vi "cam_polar.vi"(0 "camera values":T1, 2 "points":cluster{"x-point":dbl, "y-point":dbl}[](array[cluster]), 3 "camera height":sgl, 4 "Color Code":dbl) -> (6 "points polar":cluster{"degrees right":dbl, "distance":dbl}[](array[cluster]) {"degrees right" format="%#_6f"}, 7 "Angle and color of Buoys":dbl[][](array[numeric]))   [LabVIEW 2018]
panel:
  out "Array":dbl[](array[numeric])
  in  "camera angle":dbl
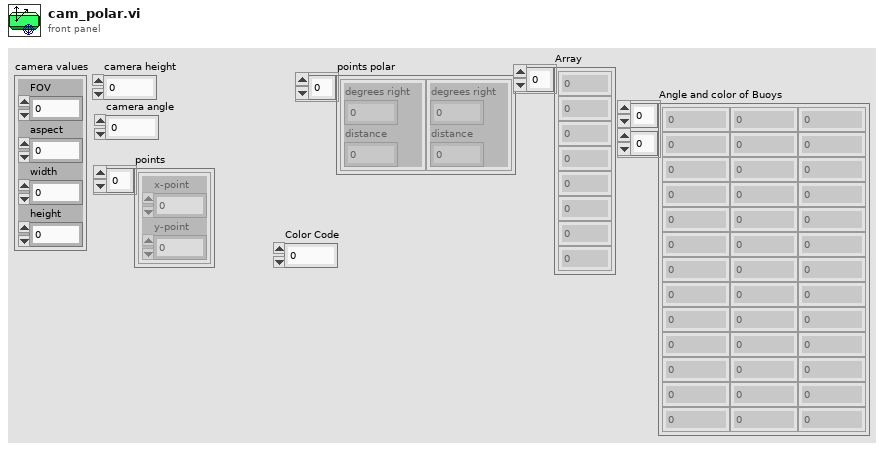
[diagram p1: front panel]
types:
  T1 = cluster{"FOV":dbl, "aspect":dbl, "width":dbl, "height":dbl}
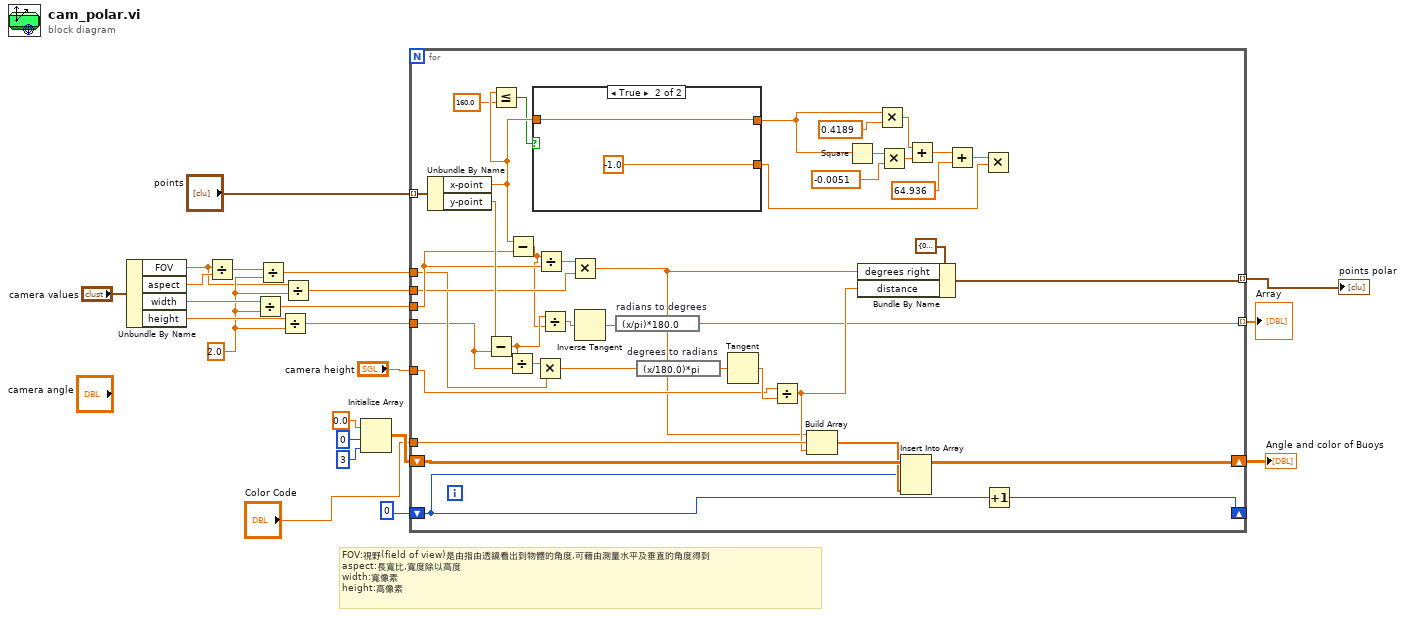
[diagram p0: block diagram]
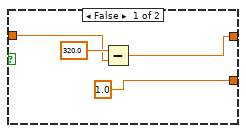
[diagram p2: hidden frame]
diagram:
  w18 = 2.0 ("y")
  # "FOV:視野(field of view)是由指由透鏡看出到物體的角度,可藉由測量水平及垂直的角度得到\naspect:長寬比,寬度除以高度\nwidth:寬像素\nheight:高像素"
  n1 = Unbundle By Name("camera values") -> ("FOV"=w2:dbl, "aspect"=w4:dbl, "width"=w20:dbl, "height"=w19:dbl)
  n2 = Divide(x=w2, y=w4) -> (x/y=w3:dbl)
  n3 = Divide(x=w20, y=w18) -> (x/y=w17:dbl)
  n4 = Divide(x=w3, y=w18) -> (x/y=w14:dbl)
  n5 = Divide(x=w19, y=w18) -> (x/y=w15:dbl)
  n6 = Divide(x=w2, y=w18) -> (x/y=w16:dbl)
  n7 = Initialize Array(0.0 ("element"), 0 ("dimension size"), 3 ("dimension size")) -> (w8:dbl[][])
  n8 = for {
    tunnel: "points" -> [w62] mode=indexing
    tunnel: w17 -> [w59]
    tunnel: w16 -> [w57]
    tunnel: w15 -> [w54]
    tunnel: w14 -> [w55]
    tunnel: [w49] -> w12 mode=indexing
    tunnel: "camera height" -> [w52]
    shift-right: [w47] -> w6
    shift-left: w8 -> [w48]
    shift-right: [w45] -> _
    shift-left: 0 ("dimension size") -> [w43]
    tunnel: "Color Code" -> [w44]
    tunnel: [w37] -> w1 mode=indexing
    n9 = Unbundle By Name(w62) -> ("x-point"=w36:dbl, "y-point"=w60:dbl)
    n10 = Subtract(x=w60, y=w54) -> (x-y=w40:dbl)
    n11 = Less Or Equal?(x=w36, y=160.0) -> (x <= y?=w24:bool)
    n12 = Divide(x=w40, y=w54) -> (x/y=w56:dbl)
    n13 = Subtract(x=w36, y=w59) -> (x-y=w39:dbl)
    n14 = case shown="True" w24 {
      tunnel: w36 -> [w64 w68]
      tunnel: [w63 w68] -> w25
      tunnel: [1.0 -1.0] -> w26
      frame False {
        n15 = Subtract(x=320.0, y=w64) -> (x-y=w63:dbl)
      }
      frame True {
      }
    }
    n16 = Multiply(x=w56, y=w55) -> (x*y=w51:dbl)
    n17 = Divide(x=w39, y=w59) -> (x/y=w58:dbl)
    n18 = Divide(x=w40, y=w39) -> (x/y=w41:dbl)
    n19 = Multiply(x=w58, y=w57) -> (x*y=w23:dbl)
    n20 = Inverse Tangent(1:w41) -> (0:w38:dbl)
    n21 = expression code="(x/pi)*180.0" "radians to degrees"(w38) -> (w37:dbl)
    n22 = expression code="(x/180.0)*pi" "degrees to radians"(w51) -> (w50:dbl)
    n23 = Tangent(1:w50) -> (0:w53:dbl)
    n24 = Divide(x=w52, y=w53) -> (x/y=w42:dbl)
    n25 = Build Array(w23, w44, w42) -> (w46:dbl[])
    n26 = Square(x=w25) -> (x^2=w28:dbl)
    n27 = Bundle By Name(cluster=cluster{"degrees right":dbl, "distance":dbl} {"degrees right"=0.0, "distance"=0.0}, "degrees right"=w23, "distance"=w42) -> (w49:cluster{"degrees right":dbl, "distance":dbl})
    n28 = Multiply(x=w25, y=0.4189) -> (x*y=w31:dbl)
    n29 = Multiply(x=w28, y=-0.0051) -> (x*y=w30:dbl)
    n30 = Insert Into Array(array=w48, index (row)=w43, new element=w46) -> (w47:dbl[][])  [unwired: 1 in]
    n31 = Add(x=w31, y=w30) -> (x+y=w33:dbl)
    n32 = Add(x=w33, y=64.936) -> (x+y=w27:dbl)
    n33 = Multiply(x=w27, y=w26) -> ()  [unwired: 1 out]
    n34 = Increment(x=w43) -> (x+1=w45:i32)
  }
  "points polar" <- w12
  "Angle and color of Buoys" <- w6
  "Array" <- w1
